vi "Autonomous Independent_old.vi"() -> ()   [LabVIEW 2012]
doc: "This VI is called when autonomous begins, and will automatically be terminated when autonomous ends. You can carry out timed or sensor driven robot movement independently without needing to return to the caller."
uses:
  Robot Global Data.vi
  <vilib>/Rock Robotics/WPI/Joystick/WPI_JoystickGetSetRefNum.vi
  <vilib>/Rock Robotics/WPI/RobotDrive/WPI_RobotDriveArcadeDrive_Standard(NoSaturation).vi
panel:
  out "S4":i32
  out "E4":i32
  out "S3":i32
  out "E3":i32
  out "S2":i32
  out "E2":i32
  out "S1":i32
  out "E1":i32
  out "Auton pitch 2":dbl(knob)=30.496220413955182 scale=0.0..50.0
  out "Auton RPM 2":dbl(knob) scale=0.0..5000.0
  in  "Auton pitch":dbl(knob)=30.496220413955182 scale=0.0..50.0
  in  "Auton RPM":dbl(knob) scale=0.0..5000.0
  in  "milliseconds to wait\nduring autonomous":u32
  in  "Desired angle to\nturn to align with feeder\nstation 2":dbl
  in  "Desired distance for\nencoder to travel straight\ntowards wall 2":dbl
  in  "Desired angle to\nturn towards wall 2":dbl
  in  "Desired distance for\nthe encoder to count 2":dbl
  in  "Desired angle to turn\nBackwards (180) 2":dbl
  in  "Autonomous Modes":T1(ring)
  in  "Desired angle to\nturn to align with feeder\nstation":dbl
  in  "Desired distance for\nencoder to travel straight\ntowards wall":dbl
  in  "Desired angle to\nturn towards wall":dbl
  in  "Desired distance for\nthe encoder to count":dbl
  in  "Desired angle to turn\nBackwards (180)":dbl
  out "Current Movement, for debugging":T2 {"Y Joystick Value" scale=1.0..-1.0; "X Joystick Value" scale=-1.0..1.0}
  in  "Array of robot movements":T3(array[cluster]) {"Y Joystick Value" scale=1.0..-1.0; "X Joystick Value" scale=-1.0..1.0}
  # "To Align With Protected Feeder Station"
  # "To Align With Unprotected Feeder Station"
  # "Be sure to right-click and choose Data Operations>>Make Current Value default if you want to save the array values with the VI"
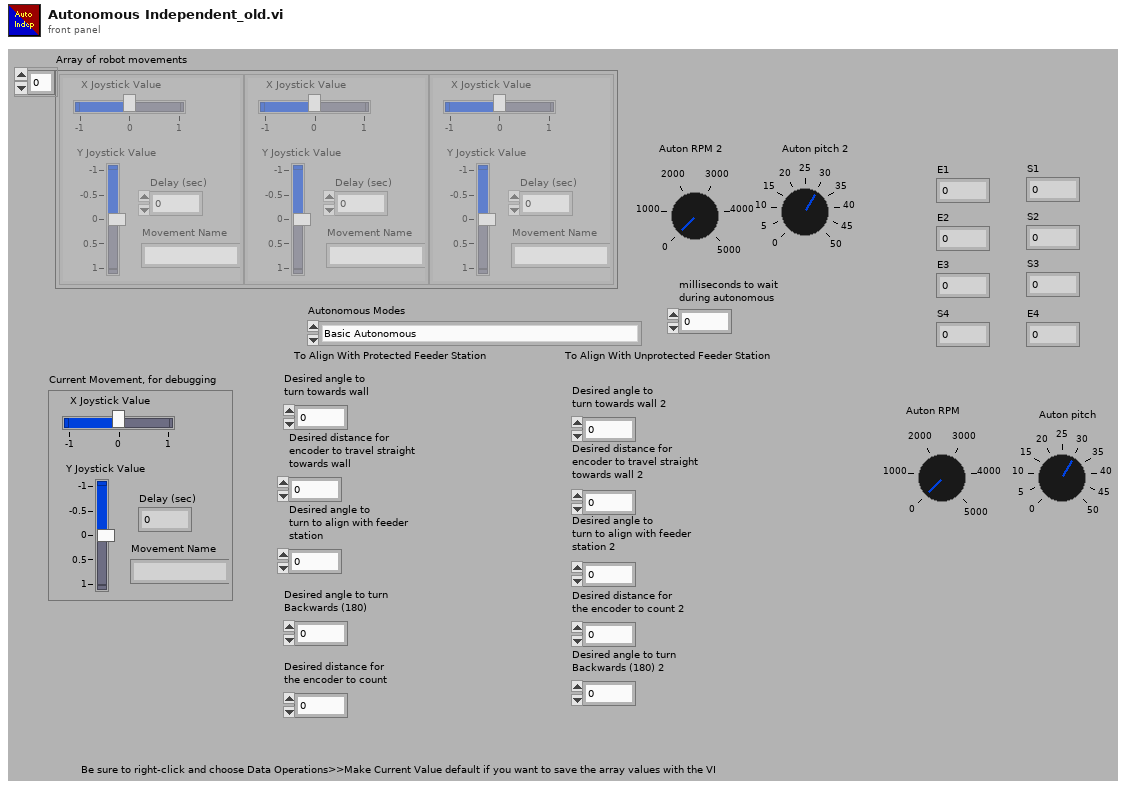
[diagram p1: front panel]
types:
  T1 = enum16{"Basic Autonomous", "Delayed Autonomous", "Shoot and Line Up With Protected Feeder Station", "Shoot and Line Up With Unprotected Feeder Station"}
  T2 = cluster{"X Joystick Value":dbl, "Y Joystick Value":dbl, "Delay (sec)":dbl, "Movement Name":string}
  T3 = cluster{"X Joystick Value":dbl, "Y Joystick Value":dbl, "Delay (sec)":dbl, "Movement Name":string}[]
  T4 = typedef "WPI_JoystickDevRef.ctl" = cluster{"Device":T5}
  T5 = typedef "WPI_JoystickDeviceEnum.ctl" = enum16{"USB 1", "USB 2", "USB 3", "USB 4", "Kinect 1", "Kinect 2"}
  T6 = cluster{"axis 1 (x)":dbl, "axis 2 (y)":dbl, "axis 3 (throttle)":dbl, "axis 4":dbl, "axis 5":dbl, "axis 6":dbl}
  T7 = typedef "WPI_RobotDriveDevRef.ctl" = cluster{"DevStatus":errorcluster, "Motors[]":T8[], "Square Inputs":bool, "Max Output":dbl, "Isochronous":bool}
  T8 = typedef "WPI_MotorControlDeviceRef.ctl" = cluster{"DeviceStatus":errorcluster, "Type":enum16{"PWM", "CAN"}, "PWM":cluster{"Digital Module":T9, "PWM Channel":T10, "DeadBand":T11}, "CAN":cluster{"Device Number":u8, "Control Mode":T12, "Semaphore":T13, "Max Vout":dbl}, "Invert":bool, "TransformRef":T14, "InvTransformRef":T14}
  T9 = typedef "FPGA_TypedefDigitalModule.ctl" = enum16{"Digital Module 1", "Digital Module 2"}
  T10 = typedef "FPGA_DIOPWMChannel.ctl" = enum8{"PWM 1", "PWM 2", "PWM 3", "PWM 4", "PWM 5", "PWM 6", "PWM 7", "PWM 8", "PWM 9", "PWM 10", "Invalid"}
  T11 = typedef "WPI_PWMDeadband.ctl" = cluster{"Name":string, "maxPositivePwm":i32, "minPositivePwm":i32, "centerPwm":i32, "maxNegativePwm":i32, "minNegativePwm":i32, "angularRange":u16}
  T12 = typedef "WPI_CANJaguar_ControlMode.ctl" = enum8{"Percent VBus", "Current", "Speed", "Position", "Voltage"}
  T13 = typedef "Semaphore RefNum" = refnum<k1>
  T14 = typedef "WPI_PWMTransform_ConPane.ctl" = refnum<vi>
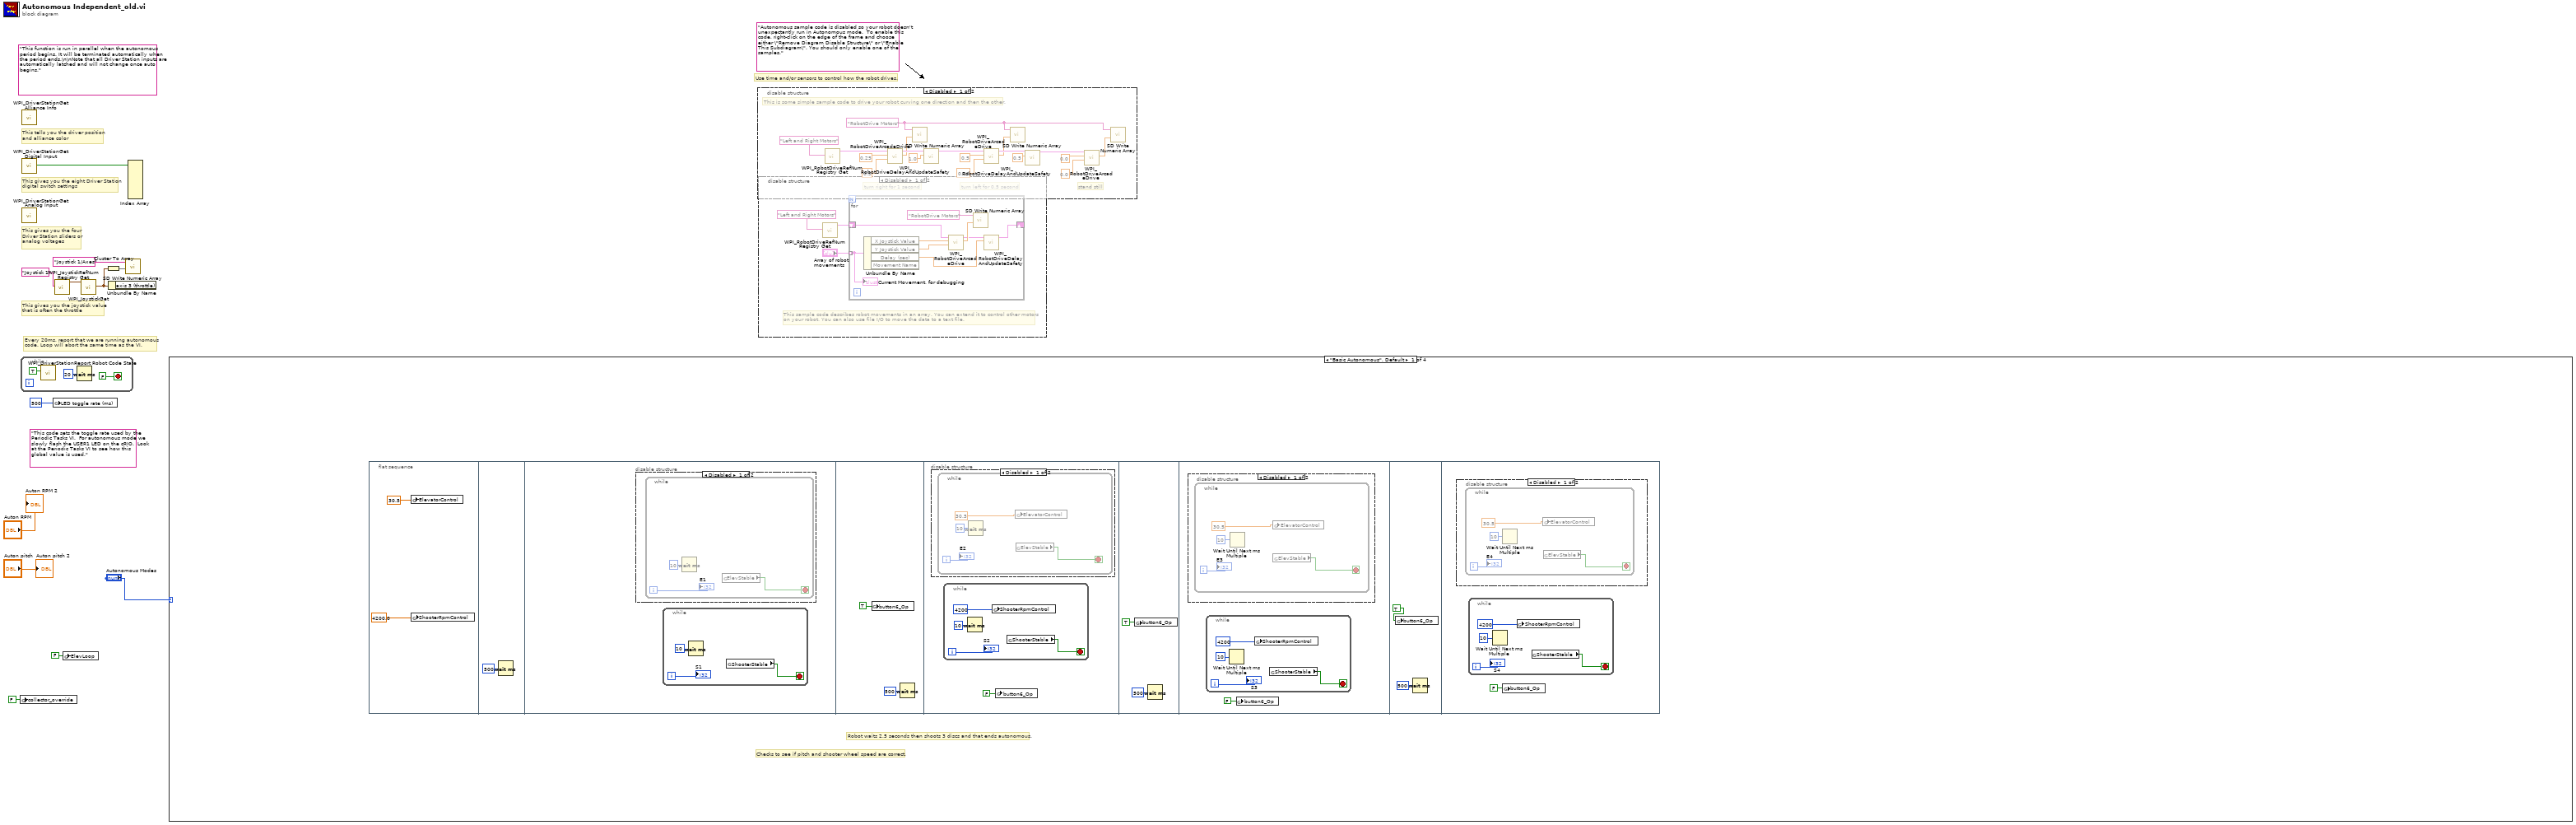
[diagram p0: block diagram]
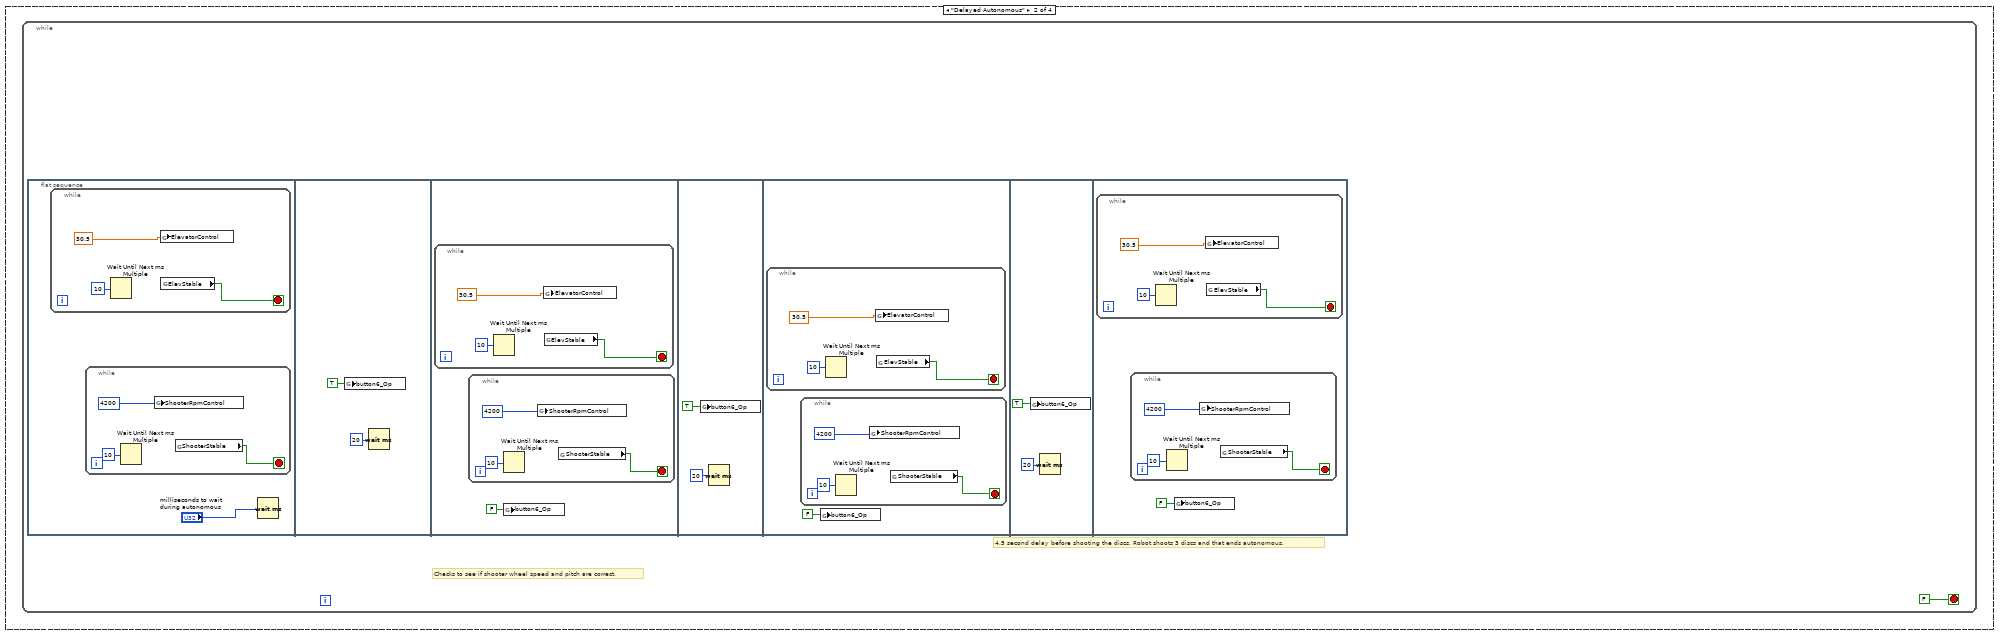
[diagram p6: hidden frame]
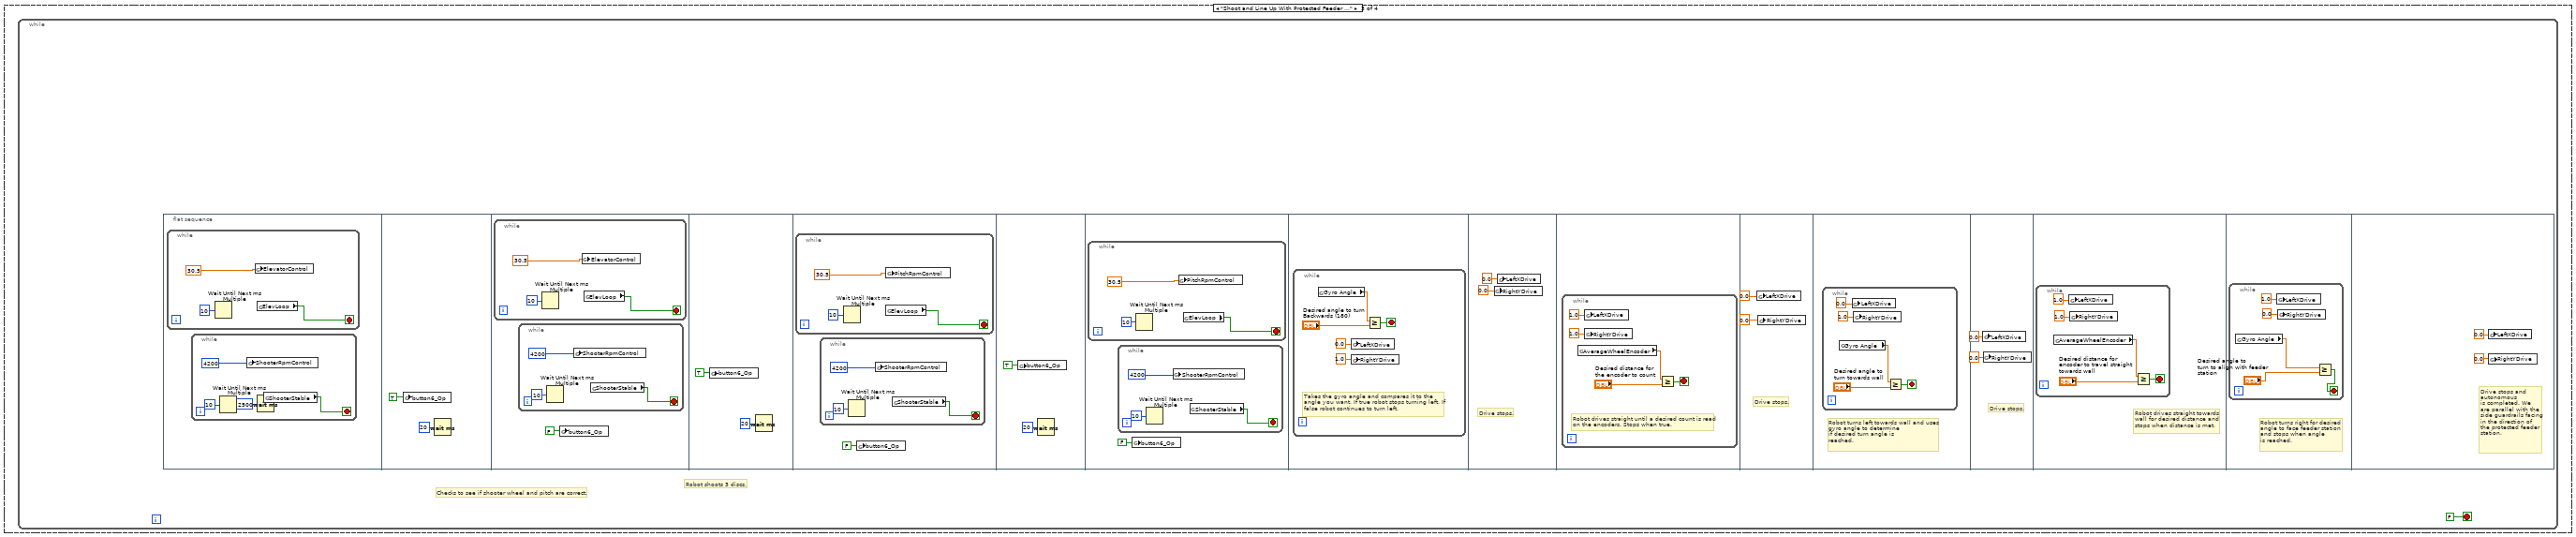
[diagram p7: hidden frame]
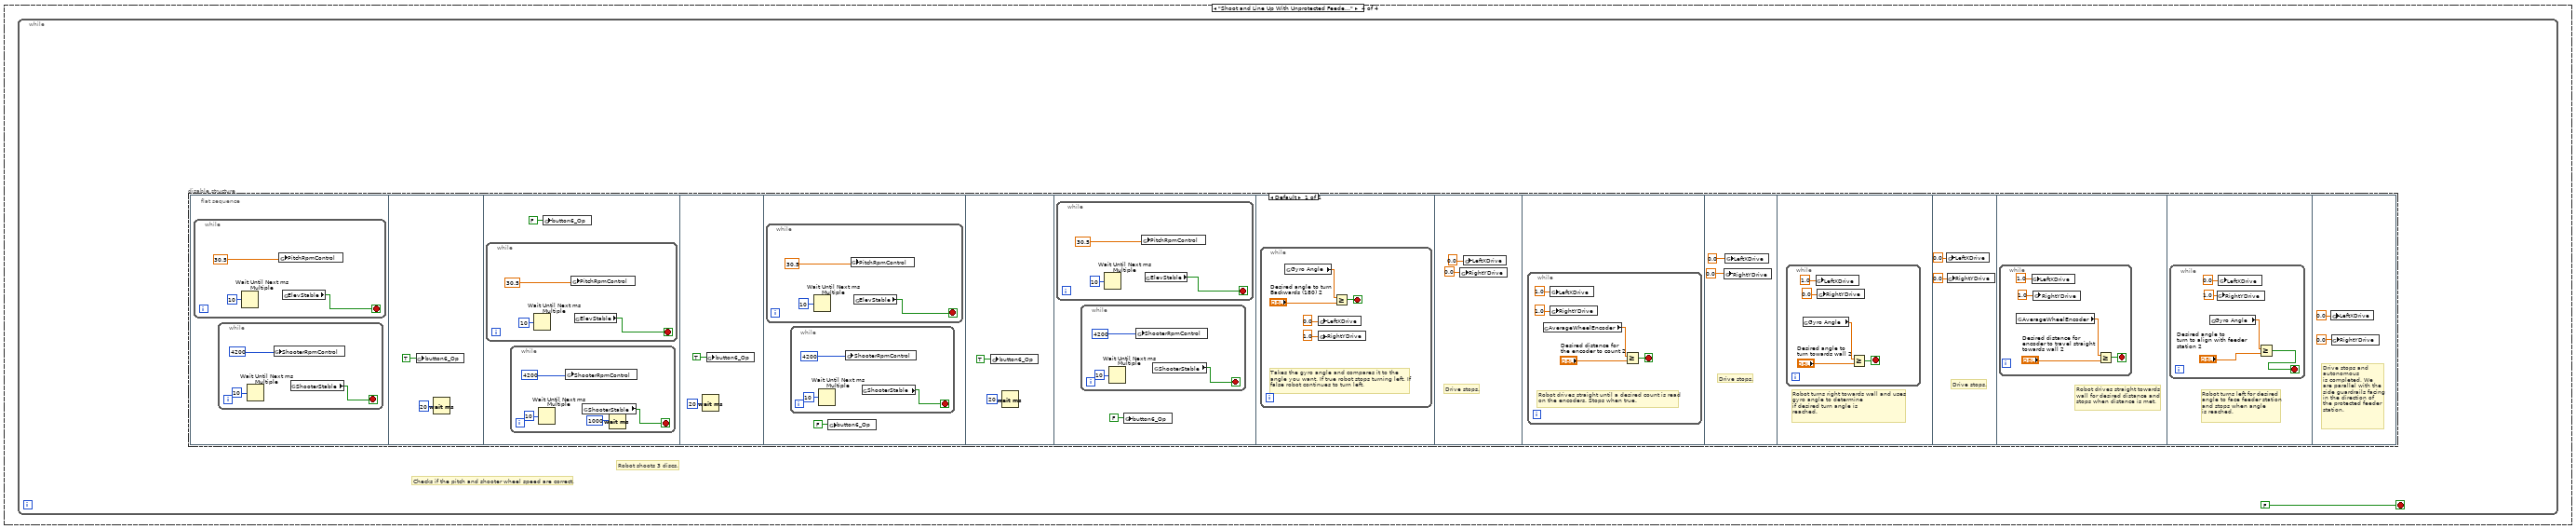
[diagram p8: hidden frame]
diagram:
  (unwired) "This code sets the toggle rate used by the Periodic Tasks VI.  For autonomous mode we slowly flash the USER1 LED on the cRIO.  Look at the Periodic Tasks VI to see how this global value is used."
  (unwired) "Autonomous sample code is disabled so your robot doesn't unexpectantly run in Autonomous mode.  To enable this code, right-click on the edge of the frame and choose either \"Remove Diagram Disable Structure\" or \"Enable This Subdiagram\". You should only enable one of the samples."
  (unwired) "This function is run in parallel when the autonomous period begins. It will be terminated automatically when the period ends.\n\nNote that all Driver Station inputs are automatically latched and will not change once auto begins."
  # "Every 20ms, report that we are running autonomous\ncode. Loop will abort the same time as the VI."
  # "This gives you the joystick value\nthat is often the throttle"
  # "Use time and/or sensors to control how the robot drives."
  # "This tells you the driver position\nand alliance color"
  # "This gives you the eight Driver Station\ndigital switch settings"
  # "This gives you the four\nDriver Station sliders or\nanalog voltages"
  n1 = global write "Robot Global Data.vi" "collector_override"(FALSE ("collector_override")) -> ()
  n2 = while {
    stop <- FALSE stop-if-true
    n3 = call <vilib>:"WPI_DriverStationReport Robot Code State.vi"("Autonomous"=TRUE) -> ()  [unwired: 10 in, 1 out]
    n4 = Wait (ms)(milliseconds to wait=u32 20) -> ()  [unwired: 1 out]
  }
  n5 = call <vilib>:"WPI_DriverStationGet Alliance Info.vi"() -> ()  [unwired: 12 out]
  n6 = call <vilib>:"WPI_DriverStationGet Digital Input.vi"() -> ("Driver Station Digital Input (1-8)"=w12:bool[])  [unwired: 11 out]
  n7 = call <vilib>:"WPI_DriverStationGet Analog Input.vi"() -> ()  [unwired: 12 out]
  n8 = global write "Robot Global Data.vi" "LED toggle rate (ms)"(u32 500 ("LED ms toggle rate")) -> ()
  n9 = call <vilib>:"WPI_JoystickRefNum Registry Get.vi"("refnum name"="Joystick 1") -> ("JoystickDevRef"=w10:T4)  [unwired: 1 in, 9 out]
  n10 = global write "Robot Global Data.vi" "ElevLoop"(FALSE ("ElevLoop")) -> ()
  n11 = call <vilib>:"WPI_JoystickGet.vi"("JoystickDevRef"=w10) -> ("Axes"=w7:T6)  [unwired: 1 in, 5 out]
  n12 = Cluster To Array(cluster=w7) -> (array=w8:dbl[])
  n13 = Unbundle By Name(w7) -> ()  [unwired: 1 out]
  n14 = call <vilib>:"SD Write Numeric Array.vi"("Numeric Array"=w8, "Name"="Joystick 1/Axes") -> ()  [unwired: 8 in, 2 out]
  n15 = Index Array(array=w12) -> ()  [unwired: 8 in, 8 out]
  n16 = case shown="\"Basic Autonomous\", Default" "Autonomous Modes" {
    frame "Basic Autonomous", Default {
      # "Checks to see if pitch and shooter wheel speed are correct."
      # "Robot waits 2.5 seconds then shoots 3 discs and that ends autonomous."
      n17 = flat-sequence {
        frame #0 {
          n18 = global write "Robot Global Data.vi" "ElevatorControl"(30.5 ("y")) -> ()
          n19 = global write "Robot Global Data.vi" "ShooterRpmControl"(4200.0 ("Value")) -> ()
        }
        frame #1 {
          n20 = Wait (ms)(milliseconds to wait=u32 500) -> ()  [unwired: 1 out]
        }
        frame #2 {
          n21 = disable-structure shown="Disabled" {
            frame Disabled {
              n22 = while {
                i -> [w19]
                stop <- w21 stop-if-true
                n23 = Wait (ms)(milliseconds to wait=u32 10 ("millisecond multiple")) -> ()  [unwired: 1 out]
                n24 = global read "Robot Global Data.vi" "ElevStable"() -> (w21:bool)
                "E1" <- w19
              }
            }
            frame Enabled {
            }
          }
          n25 = while {
            i -> [w22]
            stop <- w24 stop-if-true
            n26 = Wait (ms)(milliseconds to wait=u32 10 ("millisecond multiple")) -> ()  [unwired: 1 out]
            n27 = global read "Robot Global Data.vi" "ShooterStable"() -> (w24:bool)
            "S1" <- w22
          }
        }
        frame #3 {
          n28 = global write "Robot Global Data.vi" "button6_Op"(TRUE ("button5_Op")) -> ()
          n29 = Wait (ms)(milliseconds to wait=u32 500) -> ()  [unwired: 1 out]
        }
        frame #4 {
          n30 = disable-structure shown="Disabled" {
            frame Disabled {
              n31 = while {
                i -> [w30]
                stop <- w31 stop-if-true
                n32 = Wait (ms)(milliseconds to wait=u32 10 ("millisecond multiple")) -> ()  [unwired: 1 out]
                n33 = global write "Robot Global Data.vi" "ElevatorControl"(30.5 ("y")) -> ()
                n34 = global read "Robot Global Data.vi" "ElevStable"() -> (w31:bool)
                "E2" <- w30
              }
            }
            frame Enabled {
            }
          }
          n35 = while {
            i -> [w32]
            stop <- w34 stop-if-true
            n36 = Wait (ms)(milliseconds to wait=u32 10 ("millisecond multiple")) -> ()  [unwired: 1 out]
            n37 = global write "Robot Global Data.vi" "ShooterRpmControl"(4200 ("Value")) -> ()
            n38 = global read "Robot Global Data.vi" "ShooterStable"() -> (w34:bool)
            "S2" <- w32
          }
          n39 = global write "Robot Global Data.vi" "button6_Op"(FALSE ("button5_Op")) -> ()
        }
        frame #5 {
          n40 = global write "Robot Global Data.vi" "button6_Op"(TRUE ("button5_Op")) -> ()
          n41 = Wait (ms)(milliseconds to wait=u32 500) -> ()  [unwired: 1 out]
        }
        frame #6 {
          n42 = disable-structure shown="Disabled" {
            frame Disabled {
              n43 = while {
                i -> [w41]
                stop <- w42 stop-if-true
                n44 = Wait Until Next ms Multiple(millisecond multiple=u32 10) -> ()  [unwired: 1 out]
                n45 = global write "Robot Global Data.vi" "ElevatorControl"(30.5 ("y")) -> ()
                n46 = global read "Robot Global Data.vi" "ElevStable"() -> (w42:bool)
                "E3" <- w41
              }
            }
            frame Enabled {
            }
          }
          n47 = while {
            i -> [w43]
            stop <- w45 stop-if-true
            n48 = Wait Until Next ms Multiple(millisecond multiple=u32 10) -> ()  [unwired: 1 out]
            n49 = global write "Robot Global Data.vi" "ShooterRpmControl"(4200 ("Value")) -> ()
            n50 = global read "Robot Global Data.vi" "ShooterStable"() -> (w45:bool)
            "S3" <- w43
          }
          n51 = global write "Robot Global Data.vi" "button6_Op"(FALSE ("button5_Op")) -> ()
        }
        frame #7 {
          n52 = global write "Robot Global Data.vi" "button6_Op"(TRUE ("button5_Op")) -> ()
          n53 = Wait (ms)(milliseconds to wait=u32 500) -> ()  [unwired: 1 out]
        }
        frame #8 {
          n54 = disable-structure shown="Disabled" {
            frame Disabled {
              n55 = while {
                i -> [w50]
                stop <- w52 stop-if-true
                n56 = Wait Until Next ms Multiple(millisecond multiple=u32 10) -> ()  [unwired: 1 out]
                n57 = global write "Robot Global Data.vi" "ElevatorControl"(30.5 ("y")) -> ()
                n58 = global read "Robot Global Data.vi" "ElevStable"() -> (w52:bool)
                "E4" <- w50
              }
            }
            frame Enabled {
            }
          }
          n59 = while {
            i -> [w54]
            stop <- w56 stop-if-true
            n60 = Wait Until Next ms Multiple(millisecond multiple=u32 10) -> ()  [unwired: 1 out]
            n61 = global write "Robot Global Data.vi" "ShooterRpmControl"(4200 ("Value")) -> ()
            n62 = global read "Robot Global Data.vi" "ShooterStable"() -> (w56:bool)
            "S4" <- w54
          }
          n63 = global write "Robot Global Data.vi" "button6_Op"(FALSE ("button5_Op")) -> ()
        }
      }
    }
    frame "Delayed Autonomous" {
      n64 = while {
        stop <- FALSE stop-if-true
        # "Checks to see if shooter wheel speed and pitch are correct."
        # "4.5 second delay before shooting the discs. Robot shoots 3 discs and that ends autonomous."
        n65 = flat-sequence {
          frame #0 {
            n66 = while {
              stop <- w61 stop-if-true
              n67 = Wait Until Next ms Multiple(millisecond multiple=u32 10) -> ()  [unwired: 1 out]
              n68 = global write "Robot Global Data.vi" "ElevatorControl"(30.5 ("y")) -> ()
              n69 = global read "Robot Global Data.vi" "ElevStable"() -> (w61:bool)
            }
            n70 = while {
              stop <- w64 stop-if-true
              n71 = Wait Until Next ms Multiple(millisecond multiple=u32 10) -> ()  [unwired: 1 out]
              n72 = global write "Robot Global Data.vi" "ShooterRpmControl"(4200 ("Value")) -> ()
              n73 = global read "Robot Global Data.vi" "ShooterStable"() -> (w64:bool)
            }
            n74 = Wait (ms)(milliseconds to wait="milliseconds to wait\nduring autonomous") -> ()  [unwired: 1 out]
          }
          frame #1 {
            n75 = global write "Robot Global Data.vi" "button6_Op"(TRUE ("button5_Op")) -> ()
            n76 = Wait (ms)(milliseconds to wait=u32 20) -> ()  [unwired: 1 out]
          }
          frame #2 {
            n77 = while {
              stop <- w70 stop-if-true
              n78 = Wait Until Next ms Multiple(millisecond multiple=u32 10) -> ()  [unwired: 1 out]
              n79 = global write "Robot Global Data.vi" "ElevatorControl"(30.5 ("y")) -> ()
              n80 = global read "Robot Global Data.vi" "ElevStable"() -> (w70:bool)
            }
            n81 = while {
              stop <- w73 stop-if-true
              n82 = Wait Until Next ms Multiple(millisecond multiple=u32 10) -> ()  [unwired: 1 out]
              n83 = global write "Robot Global Data.vi" "ShooterRpmControl"(4200 ("Value")) -> ()
              n84 = global read "Robot Global Data.vi" "ShooterStable"() -> (w73:bool)
            }
            n85 = global write "Robot Global Data.vi" "button6_Op"(FALSE ("button5_Op")) -> ()
          }
          frame #3 {
            n86 = global write "Robot Global Data.vi" "button6_Op"(TRUE ("button5_Op")) -> ()
            n87 = Wait (ms)(milliseconds to wait=u32 20) -> ()  [unwired: 1 out]
          }
          frame #4 {
            n88 = while {
              stop <- w79 stop-if-true
              n89 = Wait Until Next ms Multiple(millisecond multiple=u32 10) -> ()  [unwired: 1 out]
              n90 = global write "Robot Global Data.vi" "ElevatorControl"(30.5 ("y")) -> ()
              n91 = global read "Robot Global Data.vi" "ElevStable"() -> (w79:bool)
            }
            n92 = while {
              stop <- w82 stop-if-true
              n93 = Wait Until Next ms Multiple(millisecond multiple=u32 10) -> ()  [unwired: 1 out]
              n94 = global write "Robot Global Data.vi" "ShooterRpmControl"(4200 ("Value")) -> ()
              n95 = global read "Robot Global Data.vi" "ShooterStable"() -> (w82:bool)
            }
            n96 = global write "Robot Global Data.vi" "button6_Op"(FALSE ("button5_Op")) -> ()
          }
          frame #5 {
            n97 = global write "Robot Global Data.vi" "button6_Op"(TRUE ("button5_Op")) -> ()
            n98 = Wait (ms)(milliseconds to wait=u32 20) -> ()  [unwired: 1 out]
          }
          frame #6 {
            n99 = while {
              stop <- w88 stop-if-true
              n100 = Wait Until Next ms Multiple(millisecond multiple=u32 10) -> ()  [unwired: 1 out]
              n101 = global write "Robot Global Data.vi" "ElevatorControl"(30.5 ("y")) -> ()
              n102 = global read "Robot Global Data.vi" "ElevStable"() -> (w88:bool)
            }
            n103 = while {
              stop <- w91 stop-if-true
              n104 = Wait Until Next ms Multiple(millisecond multiple=u32 10) -> ()  [unwired: 1 out]
              n105 = global write "Robot Global Data.vi" "ShooterRpmControl"(4200 ("Value")) -> ()
              n106 = global read "Robot Global Data.vi" "ShooterStable"() -> (w91:bool)
            }
            n107 = global write "Robot Global Data.vi" "button6_Op"(FALSE ("button5_Op")) -> ()
          }
        }
      }
    }
    frame "Shoot and Line Up With Protected Feeder Station" {
      n108 = while {
        stop <- FALSE stop-if-true
        # "Checks to see if shooter wheel and pitch are correct."
        # "Robot shoots 3 discs."
        n109 = flat-sequence {
          frame #0 {
            n110 = while {
              stop <- w96 stop-if-true
              n111 = Wait Until Next ms Multiple(millisecond multiple=u32 10) -> ()  [unwired: 1 out]
              n112 = global write "Robot Global Data.vi" "ElevatorControl"(30.5 ("y")) -> ()
              n113 = global read "Robot Global Data.vi" "ElevLoop"() -> (w96:bool)
            }
            n114 = while {
              stop <- w99 stop-if-true
              n115 = Wait Until Next ms Multiple(millisecond multiple=u32 10) -> ()  [unwired: 1 out]
              n116 = global write "Robot Global Data.vi" "ShooterRpmControl"(4200 ("Value")) -> ()
              n117 = global read "Robot Global Data.vi" "ShooterStable"() -> (w99:bool)
            }
            n118 = Wait (ms)(milliseconds to wait=u32 2500) -> ()  [unwired: 1 out]
          }
          frame #1 {
            n119 = global write "Robot Global Data.vi" "button6_Op"(TRUE ("button5_Op")) -> ()
            n120 = Wait (ms)(milliseconds to wait=u32 20) -> ()  [unwired: 1 out]
          }
          frame #2 {
            n121 = while {
              stop <- w105 stop-if-true
              n122 = Wait Until Next ms Multiple(millisecond multiple=u32 10) -> ()  [unwired: 1 out]
              n123 = global write "Robot Global Data.vi" "ElevatorControl"(30.5 ("y")) -> ()
              n124 = global read "Robot Global Data.vi" "ElevLoop"() -> (w105:bool)
            }
            n125 = while {
              stop <- w108 stop-if-true
              n126 = Wait Until Next ms Multiple(millisecond multiple=u32 10) -> ()  [unwired: 1 out]
              n127 = global write "Robot Global Data.vi" "ShooterRpmControl"(4200 ("Value")) -> ()
              n128 = global read "Robot Global Data.vi" "ShooterStable"() -> (w108:bool)
            }
            n129 = global write "Robot Global Data.vi" "button6_Op"(FALSE ("button5_Op")) -> ()
          }
          frame #3 {
            n130 = global write "Robot Global Data.vi" "button6_Op"(TRUE ("button5_Op")) -> ()
            n131 = Wait (ms)(milliseconds to wait=u32 20) -> ()  [unwired: 1 out]
          }
          frame #4 {
            n132 = while {
              stop <- w114 stop-if-true
              n133 = Wait Until Next ms Multiple(millisecond multiple=u32 10) -> ()  [unwired: 1 out]
              n134 = global read "Robot Global Data.vi" "ElevLoop"() -> (w114:bool)
              n135 = global write "Robot Global Data.vi" "PitchRpmControl"(30.5 ("y")) -> ()
            }
            n136 = while {
              stop <- w117 stop-if-true
              n137 = Wait Until Next ms Multiple(millisecond multiple=u32 10) -> ()  [unwired: 1 out]
              n138 = global write "Robot Global Data.vi" "ShooterRpmControl"(4200 ("Value")) -> ()
              n139 = global read "Robot Global Data.vi" "ShooterStable"() -> (w117:bool)
            }
            n140 = global write "Robot Global Data.vi" "button6_Op"(FALSE ("button5_Op")) -> ()
          }
          frame #5 {
            n141 = global write "Robot Global Data.vi" "button6_Op"(TRUE ("button5_Op")) -> ()
            n142 = Wait (ms)(milliseconds to wait=u32 20) -> ()  [unwired: 1 out]
          }
          frame #6 {
            n143 = while {
              stop <- w123 stop-if-true
              n144 = Wait Until Next ms Multiple(millisecond multiple=u32 10) -> ()  [unwired: 1 out]
              n145 = global write "Robot Global Data.vi" "PitchRpmControl"(30.5 ("y")) -> ()
              n146 = global read "Robot Global Data.vi" "ElevLoop"() -> (w123:bool)
            }
            n147 = while {
              stop <- w126 stop-if-true
              n148 = Wait Until Next ms Multiple(millisecond multiple=u32 10) -> ()  [unwired: 1 out]
              n149 = global write "Robot Global Data.vi" "ShooterRpmControl"(4200 ("Value")) -> ()
              n150 = global read "Robot Global Data.vi" "ShooterStable"() -> (w126:bool)
            }
            n151 = global write "Robot Global Data.vi" "button6_Op"(FALSE ("button5_Op")) -> ()
          }
          frame #7 {
            n152 = while {
              stop <- w132 stop-if-true
              # "Takes the gyro angle and compares it to the\nangle you want. If true robot stops turning left. If\nfalse robot continues to turn left."
              n153 = global read "Robot Global Data.vi" "Gyro Angle"() -> (w128:dbl)
              n154 = global write "Robot Global Data.vi" "LeftXDrive"(0.0 ("Left axis value")) -> ()
              n155 = global write "Robot Global Data.vi" "RightYDrive"(1.0 ("Right axis value")) -> ()
              n156 = Greater Or Equal?(x=w128, y="Desired angle to turn\nBackwards (180)") -> (x >= y?=w132:bool)
            }
          }
          frame #8 {
            # "Drive stops."
            n157 = global write "Robot Global Data.vi" "RightYDrive"(0.0 ("Right axis value")) -> ()
            n158 = global write "Robot Global Data.vi" "LeftXDrive"(0.0 ("Left axis value")) -> ()
          }
          frame #9 {
            n159 = while {
              stop <- w137 stop-if-true
              # "Robot drives straight until a desired count is read\non the encoders. Stops when true."
              n160 = global read "Robot Global Data.vi" "AverageWheelEncoder"() -> (w139:dbl)
              n161 = global write "Robot Global Data.vi" "LeftXDrive"(1.0 ("Left axis value")) -> ()
              n162 = global write "Robot Global Data.vi" "RightYDrive"(1.0 ("Right axis value")) -> ()
              n163 = Greater Or Equal?(x=w139, y="Desired distance for\nthe encoder to count") -> (x >= y?=w137:bool)
            }
          }
          frame #10 {
            # "Drive stops."
            n164 = global write "Robot Global Data.vi" "LeftXDrive"(0.0 ("LeftXDrive")) -> ()
            n165 = global write "Robot Global Data.vi" "RightYDrive"(0.0 ("LeftXDrive")) -> ()
          }
          frame #11 {
            # "Robot turns left towards wall and uses\ngyro angle to determine\nif desired turn angle is \nreached."
            n166 = while {
              stop <- w143 stop-if-true
              n167 = global read "Robot Global Data.vi" "Gyro Angle"() -> (w142:dbl)
              n168 = global write "Robot Global Data.vi" "LeftXDrive"(0.0 ("Left axis value")) -> ()
              n169 = global write "Robot Global Data.vi" "RightYDrive"(1.0 ("Right axis value")) -> ()
              n170 = Greater Or Equal?(x=w142, y="Desired angle to\nturn towards wall") -> (x >= y?=w143:bool)
            }
          }
          frame #12 {
            # "Drive stops."
            n171 = global write "Robot Global Data.vi" "LeftXDrive"(0.0 ("LeftXDrive")) -> ()
            n172 = global write "Robot Global Data.vi" "RightYDrive"(0.0 ("RightYDrive")) -> ()
          }
          frame #13 {
            # "Robot drives straight towards\nwall for desired distance and\nstops when distance is met."
            n173 = while {
              stop <- w149 stop-if-true
              n174 = global read "Robot Global Data.vi" "AverageWheelEncoder"() -> (w151:dbl)
              n175 = global write "Robot Global Data.vi" "LeftXDrive"(1.0 ("Left axis value")) -> ()
              n176 = global write "Robot Global Data.vi" "RightYDrive"(1.0 ("Right axis value")) -> ()
              n177 = Greater Or Equal?(x=w151, y="Desired distance for\nencoder to travel straight\ntowards wall") -> (x >= y?=w149:bool)
            }
          }
          frame #14 {
            # "Robot turns right for desired\nangle to face feeder station\nand stops when angle\nis reached."
            n178 = while {
              stop <- w155 stop-if-true
              n179 = global read "Robot Global Data.vi" "Gyro Angle"() -> (w154:dbl)
              n180 = global write "Robot Global Data.vi" "LeftXDrive"(1.0 ("Left axis value")) -> ()
              n181 = global write "Robot Global Data.vi" "RightYDrive"(0.0 ("Right axis value")) -> ()
              n182 = Greater Or Equal?(x=w154, y="Desired angle to\nturn to align with feeder\nstation") -> (x >= y?=w155:bool)
            }
          }
          frame #15 {
            # "Drive stops and\nautonomous\nis completed. We\nare parallel with the\nside guardrails facing\nin the direction of\nthe protected feeder\nstation."
            n183 = global write "Robot Global Data.vi" "LeftXDrive"(0.0 ("LeftXDrive")) -> ()
            n184 = global write "Robot Global Data.vi" "RightYDrive"(0.0 ("LeftXDrive")) -> ()
          }
        }
      }
    }
    frame "Shoot and Line Up With Unprotected Feeder Station" {
      n185 = while {
        stop <- FALSE stop-if-true
        # "Checks if the pitch and shooter wheel speed are correct."
        # "Robot shoots 3 discs."
        n186 = disable-structure shown="Default" {
          frame Enabled {
            n187 = flat-sequence {
              frame #0 {
                n188 = while {
                  stop <- w163 stop-if-true
                  n189 = Wait Until Next ms Multiple(millisecond multiple=u32 10) -> ()  [unwired: 1 out]
                  n190 = global write "Robot Global Data.vi" "PitchRpmControl"(30.5 ("y")) -> ()
                  n191 = global read "Robot Global Data.vi" "ElevStable"() -> (w163:bool)
                }
                n192 = while {
                  stop <- w166 stop-if-true
                  n193 = Wait Until Next ms Multiple(millisecond multiple=u32 10) -> ()  [unwired: 1 out]
                  n194 = global write "Robot Global Data.vi" "ShooterRpmControl"(4200 ("Value")) -> ()
                  n195 = global read "Robot Global Data.vi" "ShooterStable"() -> (w166:bool)
                }
              }
              frame #1 {
                n196 = global write "Robot Global Data.vi" "button6_Op"(TRUE ("button5_Op")) -> ()
                n197 = Wait (ms)(milliseconds to wait=u32 20) -> ()  [unwired: 1 out]
              }
              frame #2 {
                n198 = while {
                  stop <- w173 stop-if-true
                  n199 = Wait Until Next ms Multiple(millisecond multiple=u32 10) -> ()  [unwired: 1 out]
                  n200 = global write "Robot Global Data.vi" "PitchRpmControl"(30.5 ("y")) -> ()
                  n201 = global read "Robot Global Data.vi" "ElevStable"() -> (w173:bool)
                }
                n202 = while {
                  stop <- w176 stop-if-true
                  n203 = Wait Until Next ms Multiple(millisecond multiple=u32 10) -> ()  [unwired: 1 out]
                  n204 = global write "Robot Global Data.vi" "ShooterRpmControl"(4200 ("Value")) -> ()
                  n205 = global read "Robot Global Data.vi" "ShooterStable"() -> (w176:bool)
                }
                n206 = global write "Robot Global Data.vi" "button6_Op"(FALSE ("button5_Op")) -> ()
                n207 = Wait (ms)(milliseconds to wait=u32 1000) -> ()  [unwired: 1 out]
              }
              frame #3 {
                n208 = Wait (ms)(milliseconds to wait=u32 20) -> ()  [unwired: 1 out]
                n209 = global write "Robot Global Data.vi" "button6_Op"(TRUE ("button5_Op")) -> ()
              }
              frame #4 {
                n210 = while {
                  stop <- w182 stop-if-true
                  n211 = Wait Until Next ms Multiple(millisecond multiple=u32 10) -> ()  [unwired: 1 out]
                  n212 = global write "Robot Global Data.vi" "PitchRpmControl"(30.5 ("y")) -> ()
                  n213 = global read "Robot Global Data.vi" "ElevStable"() -> (w182:bool)
                }
                n214 = while {
                  stop <- w185 stop-if-true
                  n215 = Wait Until Next ms Multiple(millisecond multiple=u32 10) -> ()  [unwired: 1 out]
                  n216 = global write "Robot Global Data.vi" "ShooterRpmControl"(4200 ("Value")) -> ()
                  n217 = global read "Robot Global Data.vi" "ShooterStable"() -> (w185:bool)
                }
                n218 = global write "Robot Global Data.vi" "button6_Op"(FALSE ("button5_Op")) -> ()
              }
              frame #5 {
                n219 = global write "Robot Global Data.vi" "button6_Op"(TRUE ("button5_Op")) -> ()
                n220 = Wait (ms)(milliseconds to wait=u32 20) -> ()  [unwired: 1 out]
              }
              frame #6 {
                n221 = while {
                  stop <- w191 stop-if-true
                  n222 = Wait Until Next ms Multiple(millisecond multiple=u32 10) -> ()  [unwired: 1 out]
                  n223 = global write "Robot Global Data.vi" "PitchRpmControl"(30.5 ("y")) -> ()
                  n224 = global read "Robot Global Data.vi" "ElevStable"() -> (w191:bool)
                }
                n225 = while {
                  stop <- w194 stop-if-true
                  n226 = Wait Until Next ms Multiple(millisecond multiple=u32 10) -> ()  [unwired: 1 out]
                  n227 = global write "Robot Global Data.vi" "ShooterRpmControl"(4200 ("Value")) -> ()
                  n228 = global read "Robot Global Data.vi" "ShooterStable"() -> (w194:bool)
                }
                n229 = global write "Robot Global Data.vi" "button6_Op"(FALSE ("button5_Op")) -> ()
              }
              frame #7 {
                n230 = while {
                  stop <- w200 stop-if-true
                  # "Takes the gyro angle and compares it to the\nangle you want. If true robot stops turning left. If\nfalse robot continues to turn left."
                  n231 = global read "Robot Global Data.vi" "Gyro Angle"() -> (w196:dbl)
                  n232 = global write "Robot Global Data.vi" "LeftXDrive"(0.0 ("Left axis value")) -> ()
                  n233 = global write "Robot Global Data.vi" "RightYDrive"(1.0 ("Right axis value")) -> ()
                  n234 = Greater Or Equal?(x=w196, y="Desired angle to turn\nBackwards (180) 2") -> (x >= y?=w200:bool)
                }
              }
              frame #8 {
                # "Drive stops."
                n235 = global write "Robot Global Data.vi" "RightYDrive"(0.0 ("Right axis value")) -> ()
                n236 = global write "Robot Global Data.vi" "LeftXDrive"(0.0 ("Left axis value")) -> ()
              }
              frame #9 {
                n237 = while {
                  stop <- w205 stop-if-true
                  # "Robot drives straight until a desired count is read\non the encoders. Stops when true."
                  n238 = global read "Robot Global Data.vi" "AverageWheelEncoder"() -> (w207:dbl)
                  n239 = global write "Robot Global Data.vi" "LeftXDrive"(1.0 ("Left axis value")) -> ()
                  n240 = global write "Robot Global Data.vi" "RightYDrive"(1.0 ("Right axis value")) -> ()
                  n241 = Greater Or Equal?(x=w207, y="Desired distance for\nthe encoder to count 2") -> (x >= y?=w205:bool)
                }
              }
              frame #10 {
                # "Drive stops."
                n242 = global write "Robot Global Data.vi" "RightYDrive"(0.0 ("LeftXDrive")) -> ()
                n243 = global write "Robot Global Data.vi" "LeftXDrive"(0.0 ("LeftXDrive")) -> ()
              }
              frame #11 {
                # "Robot turns right towards wall and uses\ngyro angle to determine\nif desired turn angle is \nreached."
                n244 = while {
                  stop <- w211 stop-if-true
                  n245 = global read "Robot Global Data.vi" "Gyro Angle"() -> (w210:dbl)
                  n246 = global write "Robot Global Data.vi" "LeftXDrive"(1.0 ("Left axis value")) -> ()
                  n247 = global write "Robot Global Data.vi" "RightYDrive"(0.0 ("Right axis value")) -> ()
                  n248 = Greater Or Equal?(x=w210, y="Desired angle to\nturn towards wall 2") -> (x >= y?=w211:bool)
                }
              }
              frame #12 {
                # "Drive stops."
                n249 = global write "Robot Global Data.vi" "LeftXDrive"(0.0 ("LeftXDrive")) -> ()
                n250 = global write "Robot Global Data.vi" "RightYDrive"(0.0 ("RightYDrive")) -> ()
              }
              frame #13 {
                # "Robot drives straight towards\nwall for desired distance and\nstops when distance is met."
                n251 = while {
                  stop <- w217 stop-if-true
                  n252 = global read "Robot Global Data.vi" "AverageWheelEncoder"() -> (w219:dbl)
                  n253 = global write "Robot Global Data.vi" "LeftXDrive"(1.0 ("Left axis value")) -> ()
                  n254 = global write "Robot Global Data.vi" "RightYDrive"(1.0 ("Right axis value")) -> ()
                  n255 = Greater Or Equal?(x=w219, y="Desired distance for\nencoder to travel straight\ntowards wall 2") -> (x >= y?=w217:bool)
                }
              }
              frame #14 {
                # "Robot turns left for desired\nangle to face feeder station\nand stops when angle\nis reached."
                n256 = while {
                  stop <- w223 stop-if-true
                  n257 = global read "Robot Global Data.vi" "Gyro Angle"() -> (w222:dbl)
                  n258 = global write "Robot Global Data.vi" "RightYDrive"(1.0 ("Right axis value")) -> ()
                  n259 = global write "Robot Global Data.vi" "LeftXDrive"(0.0 ("Left axis value")) -> ()
                  n260 = Greater Or Equal?(x=w222, y="Desired angle to\nturn to align with feeder\nstation 2") -> (x >= y?=w223:bool)
                }
              }
              frame #15 {
                # "Drive stops and\nautonomous\nis completed. We\nare parallel with the\nside guardrails facing\nin the direction of\nthe protected feeder\nstation."
                n261 = global write "Robot Global Data.vi" "LeftXDrive"(0.0 ("LeftXDrive")) -> ()
                n262 = global write "Robot Global Data.vi" "RightYDrive"(0.0 ("LeftXDrive")) -> ()
              }
            }
          }
        }
      }
    }
  }
  n263 = disable-structure shown="Disabled" {
    frame Disabled {
      w229 = "RobotDrive Motors" ("Name")
      # "This is some simple sample code to drive your robot curving one direction and then the other."
      # "stand still"
      # "turn left for 0.5 second"
      # "turn right for 1 second"
      n264 = call <vilib>:"WPI_RobotDriveRefNum Registry Get.vi"("refnum name"="Left and Right Motors") -> ("RobotDriveDevRef"=w233:T7)  [unwired: 1 in, 9 out]
      n265 = call-poly <vilib>:"WPI_RobotDriveArcadeDrive.vi"("Y axis value"=0.5 ("X axis value"), "X axis value"=0.25, "RobotDriveDevRef"=w233) -> ("Motor Values"=w232:dbl[], "RobotDriveDevRef"=w240:T7)  [unwired: 1 in, 6 out]
      n266 = call <vilib>:"SD Write Numeric Array.vi"("Numeric Array"=w232, "Name"=w229) -> ()  [unwired: 8 in, 2 out]
      n267 = call <vilib>:"WPI_RobotDriveDelayAndUpdateSafety.vi"("Delay (s)"=1.0, "RobotDriveDevRef"=w240) -> ("RobotDriveDevRef 2"=w239:T7)  [unwired: 8 in, 1 out]
      n268 = call-poly <vilib>:"WPI_RobotDriveArcadeDrive.vi"("Y axis value"=0.25 ("X axis value"), "X axis value"=0.5, "RobotDriveDevRef"=w239) -> ("Motor Values"=w231:dbl[], "RobotDriveDevRef"=w238:T7)  [unwired: 1 in, 6 out]
      n269 = call <vilib>:"SD Write Numeric Array.vi"("Numeric Array"=w231, "Name"=w229) -> ()  [unwired: 8 in, 2 out]
      n270 = call <vilib>:"WPI_RobotDriveDelayAndUpdateSafety.vi"("Delay (s)"=0.5, "RobotDriveDevRef"=w238) -> ("RobotDriveDevRef 2"=w237:T7)  [unwired: 8 in, 1 out]
      n271 = call-poly <vilib>:"WPI_RobotDriveArcadeDrive.vi"("Y axis value"=0.0 ("X axis value"), "X axis value"=0.0, "RobotDriveDevRef"=w237) -> ("Motor Values"=w230:dbl[])  [unwired: 1 in, 7 out]
      n272 = call <vilib>:"SD Write Numeric Array.vi"("Numeric Array"=w230, "Name"=w229) -> ()  [unwired: 8 in, 2 out]
    }
    frame Enabled {
    }
  }
  n273 = disable-structure shown="Disabled" {
    frame Disabled {
      # "This sample code describes robot movements in an array. You can extend it to control other motors\non your robot. You can also use file I/O to move the data to a text file."
      n274 = call <vilib>:"WPI_RobotDriveRefNum Registry Get.vi"("refnum name"="Left and Right Motors") -> ("RobotDriveDevRef"=w248:T7)  [unwired: 1 in, 9 out]
      n275 = for {
        shift-right: [w254] -> _
        shift-left: w248 -> [w255]
        tunnel: "Array of robot movements" -> [w250] mode=indexing
        n276 = Unbundle By Name(w250) -> ("X Joystick Value"=w253:dbl, "Y Joystick Value"=w252:dbl, "Delay (sec)"=w251:dbl)  [unwired: 1 out]
        n277 = call-poly <vilib>:"WPI_RobotDriveArcadeDrive.vi"("Y axis value"=w252, "X axis value"=w253, "RobotDriveDevRef"=w255) -> ("Motor Values"=w257:dbl[], "RobotDriveDevRef"=w256:T7)  [unwired: 1 in, 6 out]
        n278 = call <vilib>:"SD Write Numeric Array.vi"("Numeric Array"=w257, "Name"="RobotDrive Motors") -> ()  [unwired: 8 in, 2 out]
        n279 = call <vilib>:"WPI_RobotDriveDelayAndUpdateSafety.vi"("Delay (s)"=w251, "RobotDriveDevRef"=w256) -> ("RobotDriveDevRef 2"=w254:T7)  [unwired: 8 in, 1 out]
        "Current Movement, for debugging" <- w250
      }
    }
    frame Enabled {
    }
  }
  "Auton RPM 2" <- "Auton RPM"
  "Auton pitch 2" <- "Auton pitch"
